vi "GetOperation.vi"(8 "Polys":T3[](array[typedef]), 9 "Crossings":T4(array[cluster]), 10 "Lines":T3, 11 "End":T5) -> (3 "Operations":T2(array[cluster]))   [LabVIEW 2014]
uses:
  TypeDefs/Point2D.ctl
  TypeDefs/Poly2D.ctl
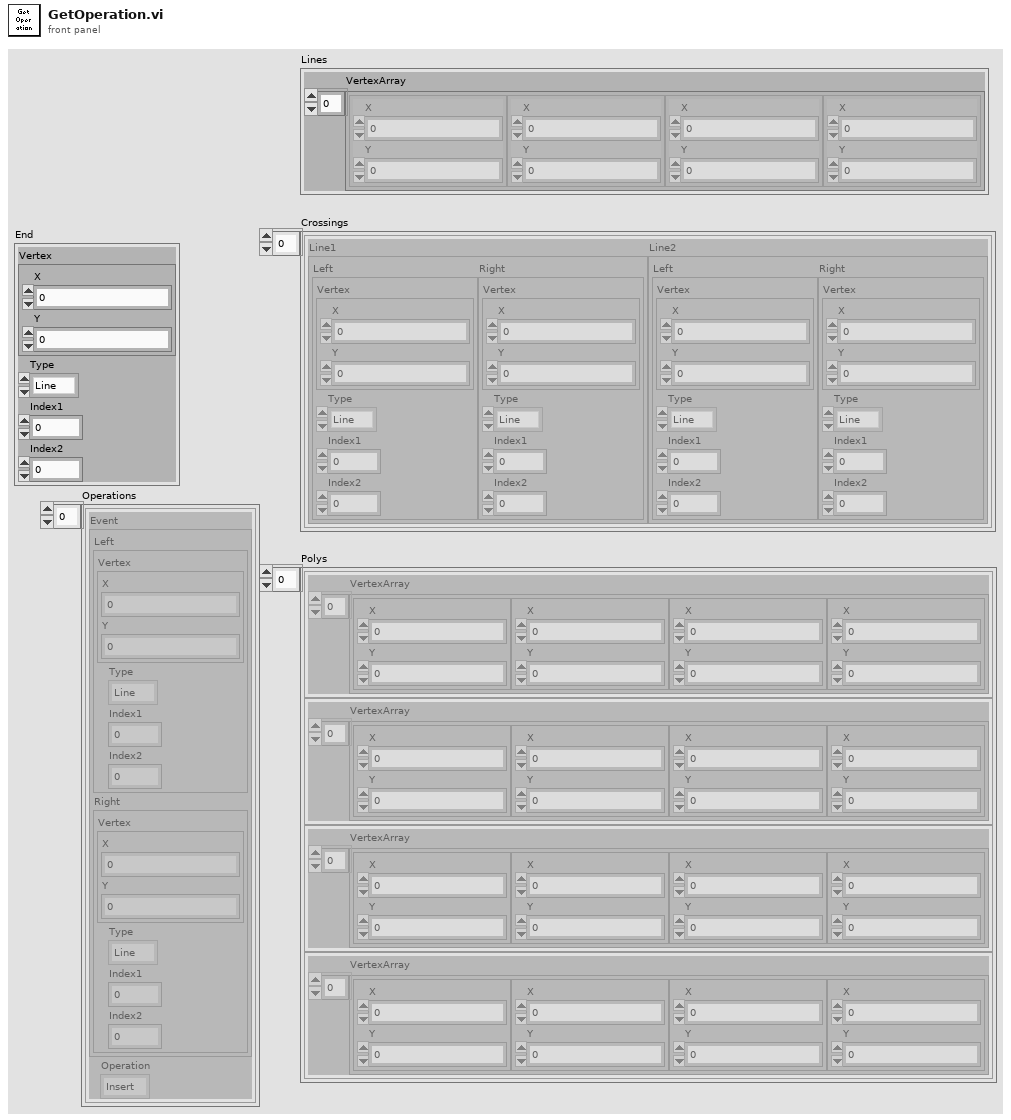
[diagram p1: front panel]
types:
  T1 = typedef "Point2D.ctl" = cluster{"X":sgl, "Y":sgl}
  T2 = cluster{"Event":cluster{"Left":cluster{"Vertex":T1, "Type":enum16{"Line", "Poly", "Cross"}, "Index1":i32, "Index2":i32}, "Right":cluster{"Vertex":T1, "Type":enum16{"Line", "Poly", "Cross"}, "Index1":i32, "Index2":i32}}, "Operation":enum16{"Insert", "Delete"}}[]
  T3 = typedef "Poly2D.ctl" = cluster{"VertexArray":T1[]}
  T4 = cluster{"Line1":cluster{"Left":cluster{"Vertex":T1, "Type":enum16{"Line", "Poly", "Cross"}, "Index1":i32, "Index2":i32}, "Right":cluster{"Vertex":T1, "Type":enum16{"Line", "Poly", "Cross"}, "Index1":i32, "Index2":i32}}, "Line2":cluster{"Left":cluster{"Vertex":T1, "Type":enum16{"Line", "Poly", "Cross"}, "Index1":i32, "Index2":i32}, "Right":cluster{"Vertex":T1, "Type":enum16{"Line", "Poly", "Cross"}, "Index1":i32, "Index2":i32}}}[]
  T5 = cluster{"Vertex":T1, "Type":enum16{"Line", "Poly", "Cross"}, "Index1":i32, "Index2":i32}
  T6 = cluster{"Event":cluster{"Left":cluster{"Vertex":T1, "Type":enum16{"Line", "Poly", "Cross"}, "Index1":i32, "Index2":i32}, "Right":cluster{"Vertex":T1, "Type":enum16{"Line", "Poly", "Cross"}, "Index1":i32, "Index2":i32}}, "Operation":enum16{"Insert", "Delete", "Swap"}}
  T7 = cluster{"Left":cluster{"Vertex":T1, "Type":enum16{"Line", "Poly", "Cross"}, "Index1":i32, "Index2":i32}, "Right":cluster{"Vertex":T1, "Type":enum16{"Line", "Poly", "Cross"}, "Index1":i32, "Index2":i32}}
  T8 = cluster{"Event":cluster{"Left":cluster{"Vertex":T1, "Type":enum16{"Line", "Poly", "Cross"}, "Index1":i32, "Index2":i32}, "Right":cluster{"Vertex":T1, "Type":enum16{"Line", "Poly", "Cross"}, "Index1":i32, "Index2":i32}}, "Operation":enum16{"Insert", "Delete", "Swap"}}[]
  T9 = cluster{"Line1":cluster{"Left":cluster{"Vertex":T1, "Type":enum16{"Line", "Poly", "Cross"}, "Index1":i32, "Index2":i32}, "Right":cluster{"Vertex":T1, "Type":enum16{"Line", "Poly", "Cross"}, "Index1":i32, "Index2":i32}}, "Line2":cluster{"Left":cluster{"Vertex":T1, "Type":enum16{"Line", "Poly", "Cross"}, "Index1":i32, "Index2":i32}, "Right":cluster{"Vertex":T1, "Type":enum16{"Line", "Poly", "Cross"}, "Index1":i32, "Index2":i32}}}
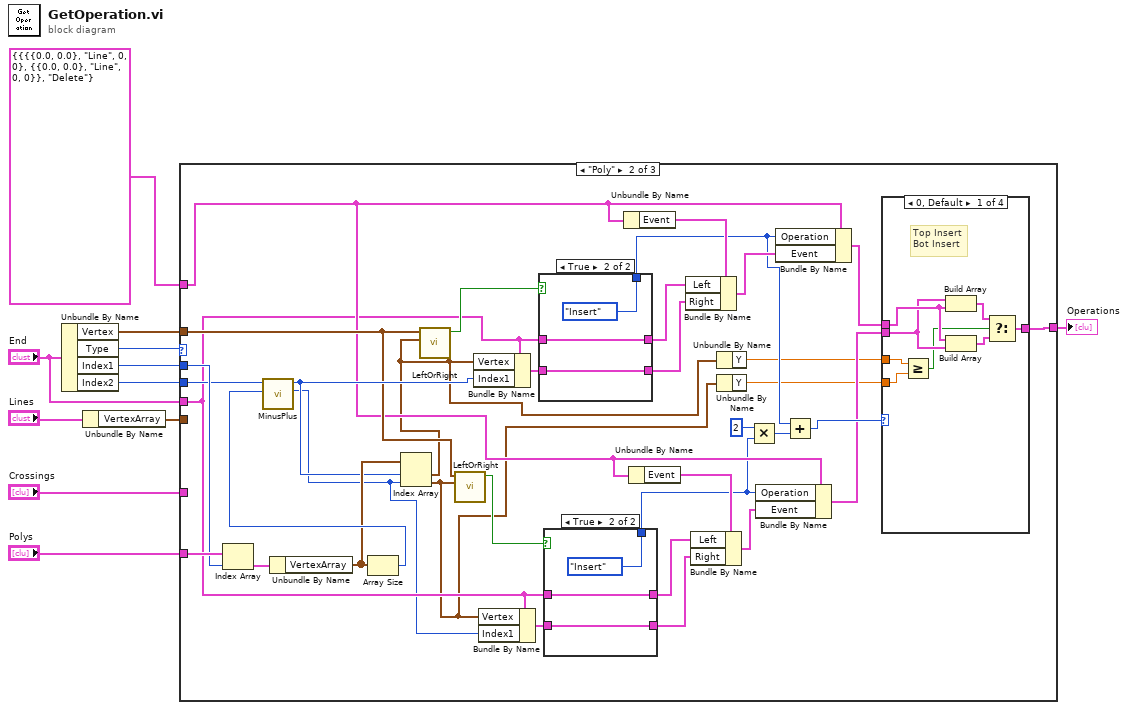
[diagram p0: block diagram]
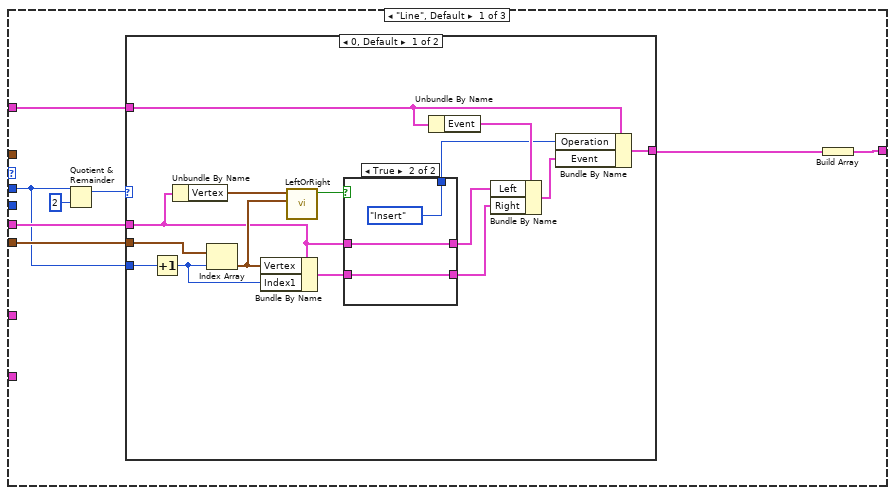
[diagram p2: hidden frame]
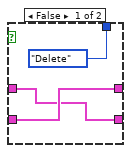
[diagram p3: hidden frame]
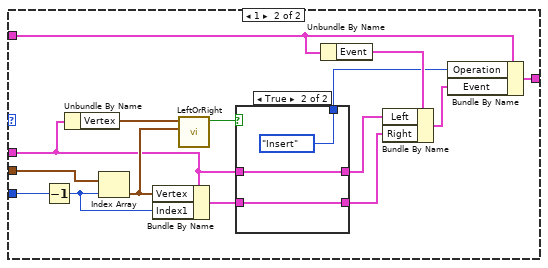
[diagram p4: hidden frame]
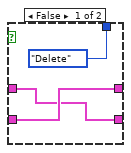
[diagram p5: hidden frame]
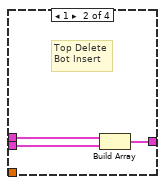
[diagram p6: hidden frame]
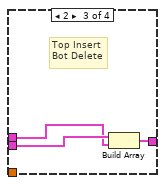
[diagram p7: hidden frame]
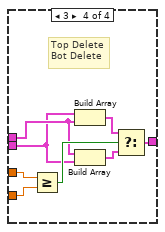
[diagram p8: hidden frame]
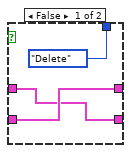
[diagram p9: hidden frame]
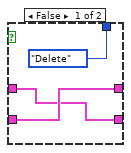
[diagram p10: hidden frame]
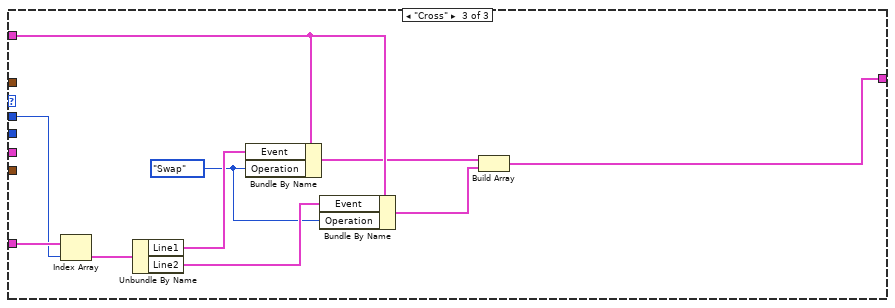
[diagram p11: hidden frame]
diagram:
  n1 = Unbundle By Name("End") -> ("Vertex"=w10:T1, "Type"=w11:enum16{"Line", "Poly", "Cross"}, "Index1"=w9:i32, "Index2"=w8:i32)
  n2 = Unbundle By Name("Lines") -> ("VertexArray"=w4:T1[])
  n3 = case shown="\"Poly\"" w11 {
    tunnel: w10 -> [_ w83 _]
    tunnel: w9 -> [w14 w95 w139]
    tunnel: w8 -> [_ w93 _]
    tunnel: w4 -> [w15 _ _]
    tunnel: T6 {"Event"={"Left"={"Vertex"={"X"=0.0, "Y"=0.0}, "Type"=enum."Line", "Index1"=0, "Index2"=0}, "Right"={"Vertex"={"X"=0.0, "Y"=0.0}, "Type"=enum."Line", "Index1"=0, "Index2"=0}}, "Operation"=enum."Delete"} -> [w17 w76 w135]
    tunnel: "End" -> [w16 w75 _]
    tunnel: [w13 w66 w131] -> w2
    tunnel: "Polys" -> [_ w96 _]
    tunnel: "Crossings" -> [_ _ w140]
    frame "Line", Default {
      n4 = Quotient & Remainder(x=w14, y=2) -> (x-y*floor(x/y)=w18:i32)  [unwired: 1 out]
      n5 = case shown="0, Default" w18 {
        tunnel: w17 -> [w34 w45]
        tunnel: w16 -> [w23 w41]
        tunnel: w15 -> [w30 w44]
        tunnel: w14 -> [w31 w42]
        tunnel: [w28 w43] -> w12
        frame 0, Default {
          n6 = Increment(x=w31) -> (x+1=w29:i32)
          n7 = Unbundle By Name(w23) -> ("Vertex"=w27:T1)
          n8 = Index Array(array=w30, index=w29) -> (element=w26:T1)
          n9 = Bundle By Name(cluster=w23, "Vertex"=w26, "Index1"=w29) -> (w21:T5)
          n10 = call "LeftOrRight.vi"("Vertex2"=w26, "Vertex1"=w27) -> ("Left/Right"=w25:bool)  [unwired: 9 in]
          n11 = case shown="True" w25 {
            tunnel: [w37 w40] -> w24
            tunnel: w23 -> [w36 w40]
            tunnel: [w36 w39] -> w22
            tunnel: w21 -> [w37 w39]
            tunnel: [enum16{"Insert", "Delete"}."Delete" ("Operation") enum16{"Insert", "Delete"}."Insert" ("Operation")] -> w20
            frame False {
            }
            frame True {
            }
          }
          n12 = Unbundle By Name(w34) -> ("Event"=w33:T7)
          n13 = Bundle By Name(cluster=w33, "Left"=w24, "Right"=w22) -> (w32:T7)
          n14 = Bundle By Name(cluster=w34, "Operation"=w20, "Event"=w32) -> (w28:T6)
        }
        frame 1 {
          n15 = Decrement(x=w42) -> (x-1=w53:i32)
          n16 = Unbundle By Name(w41) -> ("Vertex"=w52:T1)
          n17 = Index Array(array=w44, index=w53) -> (element=w51:T1)
          n18 = Bundle By Name(cluster=w41, "Vertex"=w51, "Index1"=w53) -> (w47:T5)
          n19 = call "LeftOrRight.vi"("Vertex2"=w51, "Vertex1"=w52) -> ("Left/Right"=w50:bool)  [unwired: 9 in]
          n20 = case shown="True" w50 {
            tunnel: [w58 w61] -> w49
            tunnel: w41 -> [w57 w61]
            tunnel: [w57 w60] -> w48
            tunnel: w47 -> [w58 w60]
            tunnel: [enum16{"Insert", "Delete"}."Delete" ("Operation") enum16{"Insert", "Delete"}."Insert" ("Operation")] -> w46
            frame False {
            }
            frame True {
            }
          }
          n21 = Unbundle By Name(w45) -> ("Event"=w55:T7)
          n22 = Bundle By Name(cluster=w55, "Left"=w49, "Right"=w48) -> (w54:T7)
          n23 = Bundle By Name(cluster=w45, "Operation"=w46, "Event"=w54) -> (w43:T6)
        }
      }
      n24 = Build Array(w12) -> (w13:T8)
    }
    frame "Poly" {
      n25 = Index Array(array=w96, index=w95) -> (element=w94:T3)
      n26 = Unbundle By Name(w94) -> ("VertexArray"=w91:T1[])
      n27 = Array Size(array=w91) -> (size(s)=w92:i32)
      n28 = call "MinusPlus.vi"("Wrap"=w92, "Index"=w93) -> ("Plus"=w74:i32, "Minus"=w84:i32)  [unwired: 8 in]
      n29 = Index Array(array=w91, index #1=w84, index #2=w74) -> (element #1=w65:T1, element #2=w64:T1)
      n30 = call "LeftOrRight.vi"("Vertex2"=w65, "Vertex1"=w83) -> ("Left/Right"=w86:bool)  [unwired: 9 in]
      n31 = call "LeftOrRight.vi"("Vertex2"=w64, "Vertex1"=w83) -> ("Left/Right"=w77:bool)  [unwired: 9 in]
      n32 = Bundle By Name(cluster=w75, "Vertex"=w65, "Index1"=w84) -> (w85:T5)
      n33 = Bundle By Name(cluster=w75, "Vertex"=w64, "Index1"=w74) -> (w82:T5)
      n34 = case shown="True" w86 {
        tunnel: [w127 w130] -> w88
        tunnel: w75 -> [w126 w130]
        tunnel: [w126 w129] -> w87
        tunnel: w85 -> [w127 w129]
        tunnel: [enum16{"Insert", "Delete"}."Delete" ("Operation") enum16{"Insert", "Delete"}."Insert" ("Operation")] -> w70
        frame False {
        }
        frame True {
        }
      }
      n35 = case shown="True" w77 {
        tunnel: [w121 w124] -> w80
        tunnel: w75 -> [w120 w124]
        tunnel: [w120 w123] -> w81
        tunnel: w82 -> [w121 w123]
        tunnel: [enum16{"Insert", "Delete"}."Delete" ("Operation") enum16{"Insert", "Delete"}."Insert" ("Operation")] -> w73
        frame False {
        }
        frame True {
        }
      }
      n36 = Unbundle By Name(w76) -> ("Event"=w90:T7)
      n37 = Unbundle By Name(w76) -> ("Event"=w78:T7)
      n38 = Bundle By Name(cluster=w90, "Left"=w88, "Right"=w87) -> (w89:T7)
      n39 = Bundle By Name(cluster=w78, "Left"=w80, "Right"=w81) -> (w79:T7)
      n40 = Unbundle By Name(w65) -> ("Y"=w63:sgl)
      n41 = Unbundle By Name(w64) -> ("Y"=w62:sgl)
      n42 = Multiply(x=2, y=w73) -> (x*y=w71:i32)
      n43 = Bundle By Name(cluster=w76, "Operation"=w73, "Event"=w79) -> (w67:T6)
      n44 = Bundle By Name(cluster=w76, "Operation"=w70, "Event"=w89) -> (w68:T6)
      n45 = Add(x=w70, y=w71) -> (x+y=w69:i32)
      n46 = case shown="0, Default" w69 {
        tunnel: w68 -> [w102 w107 w108 w115]
        tunnel: w67 -> [w101 w106 w109 w114]
        tunnel: [w97 w105 w110 w111] -> w66
        tunnel: w63 -> [w104 _ _ w113]
        tunnel: w62 -> [w103 _ _ w112]
        frame 0, Default {
          # "Top Insert\nBot Insert"
          n47 = Greater Or Equal?(x=w104, y=w103) -> (x >= y?=w98:bool)
          n48 = Build Array(w101, w102) -> (w100:T8)
          n49 = Build Array(w102, w101) -> (w99:T8)
          n50 = Select(t=w100, s=w98, f=w99) -> (s? t:f=w97:T8)
        }
        frame 1 {
          # "Top Delete\nBot Insert"
          n51 = Build Array(w107, w106) -> (w105:T8)
        }
        frame 2 {
          # "Top Insert\nBot Delete"
          n52 = Build Array(w109, w108) -> (w110:T8)
        }
        frame 3 {
          # "Top Delete\nBot Delete"
          n53 = Greater Or Equal?(x=w113, y=w112) -> (x >= y?=w116:bool)
          n54 = Build Array(w114, w115) -> (w118:T8)
          n55 = Build Array(w115, w114) -> (w117:T8)
          n56 = Select(t=w118, s=w116, f=w117) -> (s? t:f=w111:T8)
        }
      }
    }
    frame "Cross" {
      w134 = enum16{"Insert", "Delete", "Swap"}."Swap" ("Operation")
      n57 = Index Array(array=w140, index=w139) -> (element=w138:T9)
      n58 = Unbundle By Name(w138) -> ("Line1"=w137:T7, "Line2"=w136:T7)
      n59 = Bundle By Name(cluster=w135, "Event"=w137, "Operation"=w134) -> (w133:T6)
      n60 = Bundle By Name(cluster=w135, "Event"=w136, "Operation"=w134) -> (w132:T6)
      n61 = Build Array(w133, w132) -> (w131:T8)
    }
  }
  "Operations" <- w2
